vi "pco.camera_SaveImages_Example_IMAQ.vi"() -> ()   [LabVIEW 2020]
uses:
  <userlib>/PCO LabVIEW 5.0.0/pco.camera/Camera.lvclass
panel:
  out "rawImage":u16[][](array[numeric])
  out "Image":T1(plugin-control)
  in  "data_format":T2(ring)=enum."Mono16"
  in  "Image Index":u32 max=9
  in  "saveImages":bool
  in  "SavePath":path
  out "Recorded Images":u32
  in  "Quit":bool
  in  "roiY1":u64=2 min=2 max=2160 step=1
  in  "roiX1":u64=2 min=2 max=2560 step=1
  in  "roiY0":u64=1 min=1 max=2159 step=1
  in  "roiX0":u64=1 min=1 max=2559 step=1
  out "Image Height":u16
  out "Image Width":u16
  in  "dwImgCount":u32=10 caption="Required Number of Images" max=4023
  out "Error":errorcluster {"code" format="%x"}
  # "This example shows how to record an image sequence and save all images to files (and an .avi) afterwards.\nIt is a good starting point for writing own applications with file saving\nBut it will not be fail save, i.e. doesnt react on errors, just handles them forward to the end\n\nUsage:\nSelect your required image count you want to record before you start the program.\nOnce started, the camera class will be initialized and images will be recorded automatically.\nWhen acquisition has finished you can read the images by index, crop them using the ROI parameters and select a file path.\nBy clicking save, the images are saved with the selected file format using the current active roi setting.\nThis also finishes the program and will force an exit of the camera class"
  # "pco.labview"
  # "Camera Setup"
  # "Recording Control"
  # "Parameters for image readout"
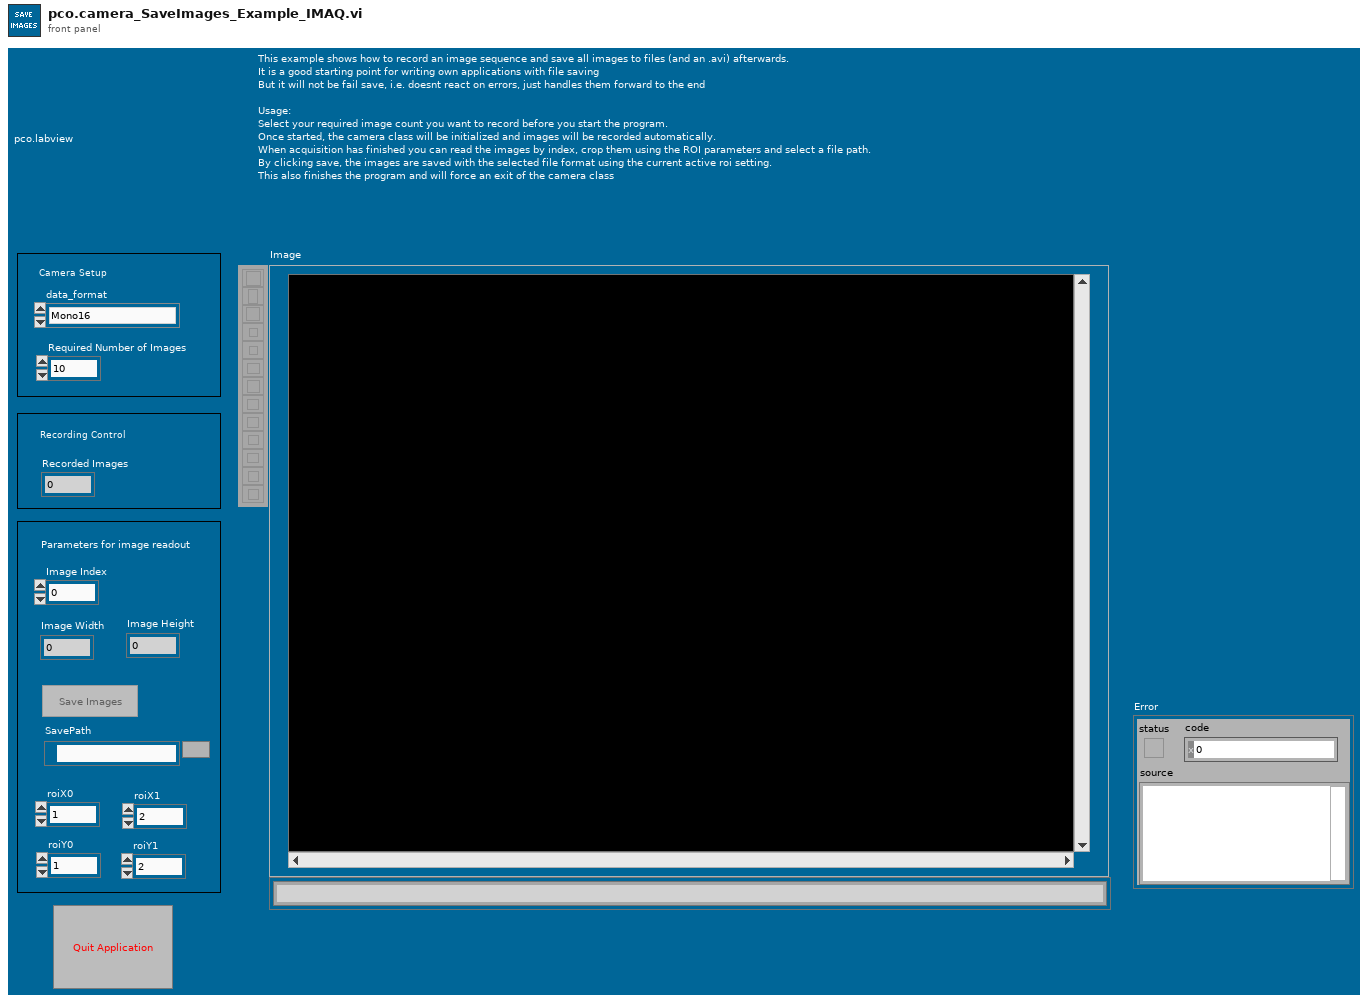
[diagram p1: front panel]
types:
  T1 = typedef "IMAQ Image.ctl" = refnum<image>
  T2 = enum16{"Undefined", "Mono8", "Mono16", "BGRA8", "RGBA8", "BGRA16", "RGBA16", "CompressedMono8"}
  T3 = enum8{"Enabled", "Disabled", "Disabled and Grayed Out"}
  T4 = enum16{"sequence", "sequence non blocking", "ring buffer", "fifo", "sequence_dpcore", "sequence_non_blocking_dpcore", "ring_buffer_dpcore", "fifo_dpcore", "tif", "multitif", "pcoraw", "b16", "dicom", "multidicom"}
  T5 = typedef "Image Type" = u32
  T6 = typedef "Camera.lvclass/binning.ctl" = cluster{"vert":u16, "horz":u16}
  T7 = cluster{"exposure_time_s":dbl, "delay_time_s":dbl, "roi":cluster{"x0":u64, "y0":u64, "x1":u64, "y1":u64}, "timestamp_mode":u16, "pixelrate":u32, "trigger_mode":u16, "acquire_mode":u16, "metadata_mode":u16, "noisefilter_mode":u16, "binning":T6}
  T8 = typedef "Color (U64)" = cluster{"Plane 3 (Blue)":u16, "Plane 2 (Green)":u16, "Plane 1 (Red)":u16, "Plane 4 (alpha)":u16}
  T9 = cluster{"dwImgCounter":u32, "lvTimestamp":timestamp, "dwMicroSeconds":u32}[]
  T10 = cluster{"dwImgCounter":u32, "lvTimestamp":timestamp, "dwMicroSeconds":u32}
  T11 = typedef "IMAQ AVI2 Refnum.ctl" = refnum<k20>
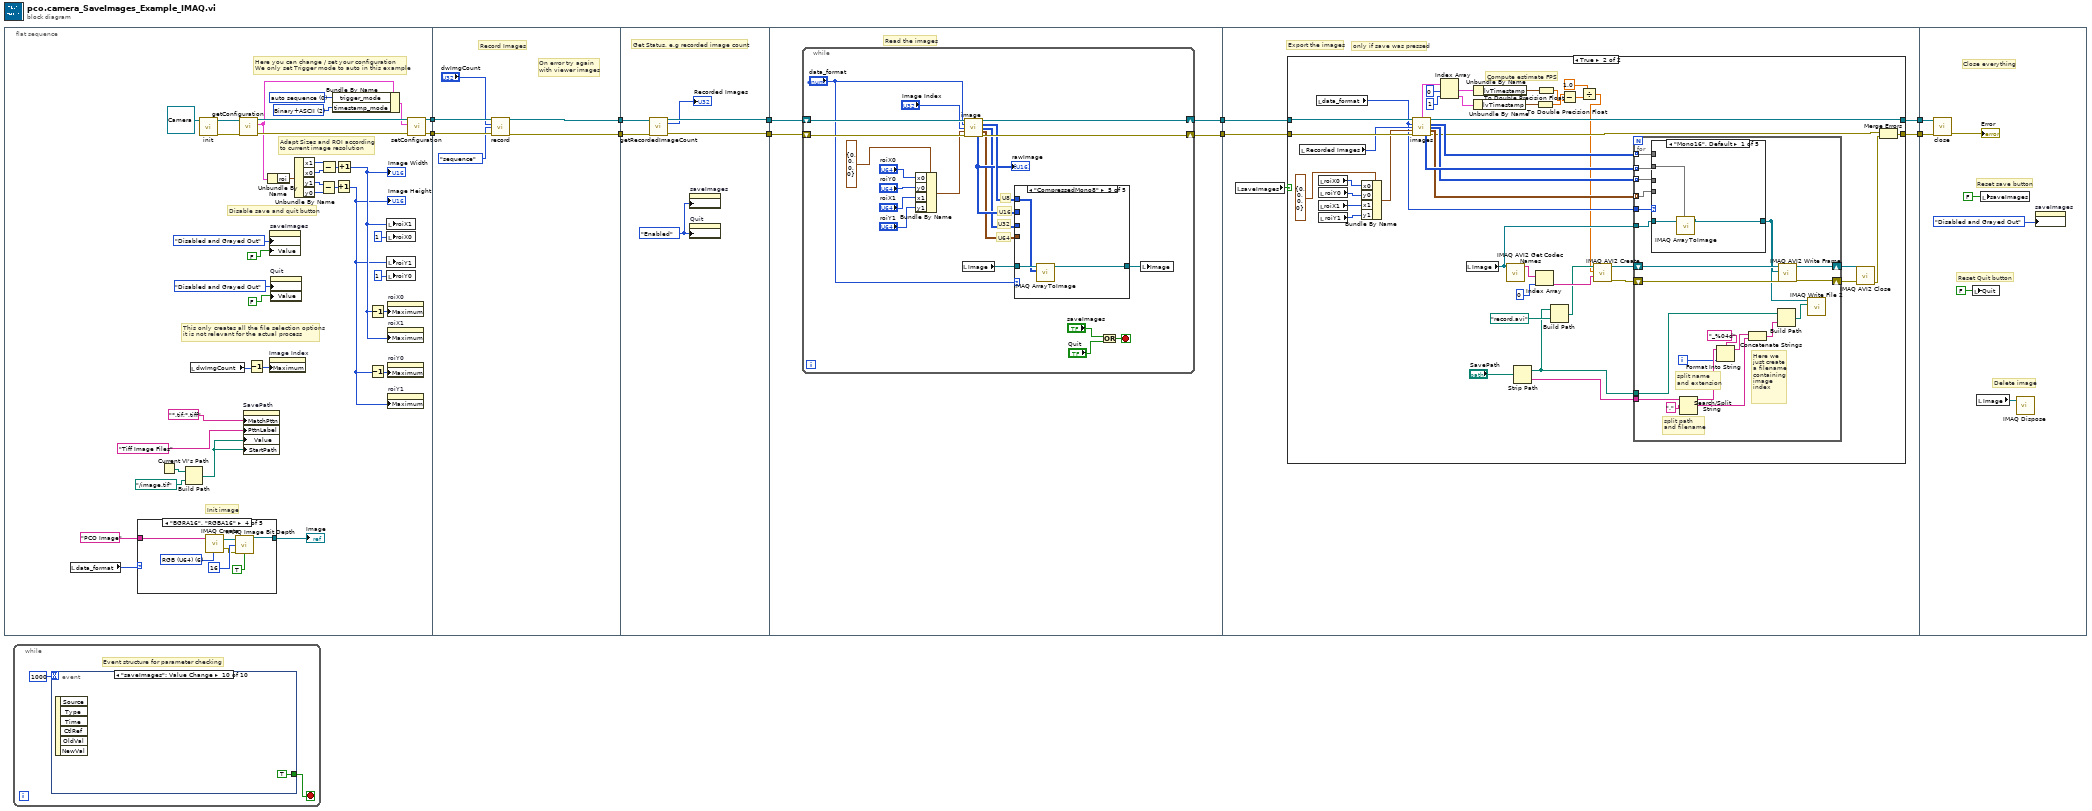
[diagram p0: block diagram]
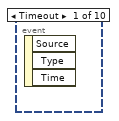
[diagram p2: hidden frame]
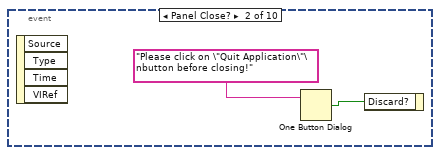
[diagram p3: hidden frame]
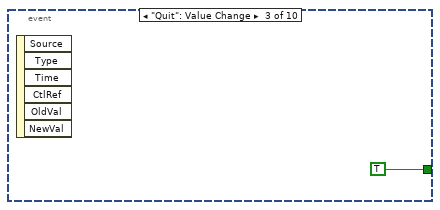
[diagram p4: hidden frame]
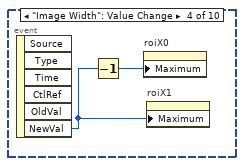
[diagram p5: hidden frame]
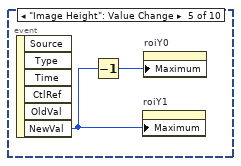
[diagram p6: hidden frame]
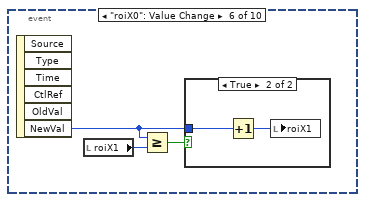
[diagram p7: hidden frame]
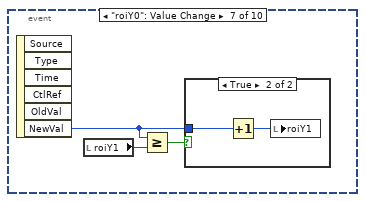
[diagram p9: hidden frame]
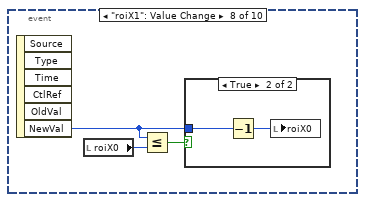
[diagram p11: hidden frame]
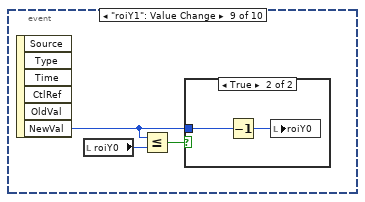
[diagram p13: hidden frame]
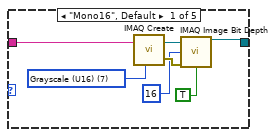
[diagram p15: hidden frame]
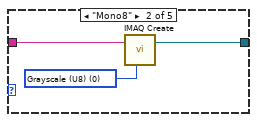
[diagram p16: hidden frame]
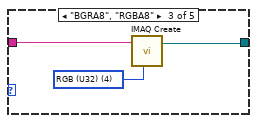
[diagram p17: hidden frame]
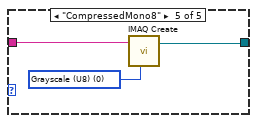
[diagram p18: hidden frame]
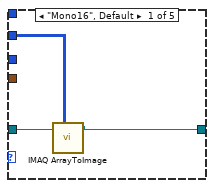
[diagram p19: hidden frame]
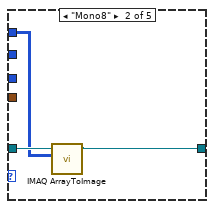
[diagram p20: hidden frame]
diagram:
  n1 = flat-sequence {
    tunnel: [w39] -> w10
    tunnel: [w38] -> w9
    tunnel: w10 -> [w77]
    tunnel: w9 -> [w76]
    tunnel: [w74] -> w8
    tunnel: [w73] -> w7
    tunnel: w8 -> [w83]
    tunnel: w7 -> [w82]
    tunnel: [w81] -> w6
    tunnel: [w80] -> w5
    tunnel: w6 -> [w86]
    tunnel: w5 -> [w87]
    tunnel: [w85] -> w4
    tunnel: [w84] -> w2
    tunnel: w4 -> [w127]
    tunnel: [w126] -> w3
    tunnel: w2 -> [w125]
    tunnel: [w124] -> w1
    tunnel: w3 -> [w216]
    tunnel: w1 -> [w215]
    frame #0 {
      w23 = u16 2 items=["OFF", "Binary", "Binary+ASCII", "ASCII"] ("TimestampMode")
      w45 = u16 0 items=["auto sequence"=0, "software trigger"=1, "external exposure start & software trigger"=2, "external exposure control"=3, "external synchronized"=4, "fast external exposure control"=5, "external CDS control"=6, "slow external exposure control"=7, "external synchronized HDSDI"=258] ("TriggerMode")
      # "Init image"
      # "This only creates all the file selection options\nit is not relevant for the actual process"
      # "Adapt Sizes and ROI according\nto current image resolution"
      # "Disable save and quit button"
      # "Here you can change / set your configuration\nWe only set Trigger mode to auto in this example"
      n2 = local read "data_format"() -> (w13:T2)
      n3 = case shown="\"BGRA16\", \"RGBA16\"" w13 {
        tunnel: "PCO Image" ("Image Name") -> [w54 w58 w60 w67 w70]
        tunnel: [w49 w56 w59 w64 w69] -> w12
        frame "Mono16", Default {
          w55 = T5 7 items=["Grayscale (U8)", "Grayscale (I16)", "Grayscale (SGL)", "Complex (CSG)", "RGB (U32)", "HSL (U32)", "RGB (U64)", "Grayscale (U16)"] ("Image Type")
          n4 = call "IMAQ Create"("Image Name"=w54, "Image Type"=w55) -> ("New Image"=w53:T1, "error out"=w52:errorcluster)  [unwired: 3 in]
          n5 = call "IMAQ Image Bit Depth"("Image"=w53, "Bit Depth (0)"=u32 16, "error in (no error)"=w52, "Get/Set Bit Depth? (Set)"=TRUE) -> ("Image Out"=w49:T1)  [unwired: 9 in, 2 out]
        }
        frame "Mono8" {
          w57 = T5 0 items=["Grayscale (U8)", "Grayscale (I16)", "Grayscale (SGL)", "Complex (CSG)", "RGB (U32)", "HSL (U32)", "RGB (U64)", "Grayscale (U16)"] ("Image Type")
          n6 = call "IMAQ Create"("Image Name"=w58, "Image Type"=w57) -> ("New Image"=w56:T1)  [unwired: 3 in, 1 out]
        }
        frame "BGRA8", "RGBA8" {
          w61 = T5 4 items=["Grayscale (U8)", "Grayscale (I16)", "Grayscale (SGL)", "Complex (CSG)", "RGB (U32)", "HSL (U32)", "RGB (U64)", "Grayscale (U16)"] ("Image Type")
          n7 = call "IMAQ Create"("Image Name"=w60, "Image Type"=w61) -> ("New Image"=w59:T1)  [unwired: 3 in, 1 out]
        }
        frame "BGRA16", "RGBA16" {
          w68 = T5 6 items=["Grayscale (U8)", "Grayscale (I16)", "Grayscale (SGL)", "Complex (CSG)", "RGB (U32)", "HSL (U32)", "RGB (U64)", "Grayscale (U16)"] ("Image Type")
          n8 = call "IMAQ Create"("Image Name"=w67, "Image Type"=w68) -> ("New Image"=w65:T1, "error out"=w62:errorcluster)  [unwired: 3 in]
          n9 = call "IMAQ Image Bit Depth"("Image"=w65, "Bit Depth (0)"=u32 16, "error in (no error)"=w62, "Get/Set Bit Depth? (Set)"=TRUE) -> ("Image Out"=w64:T1)  [unwired: 9 in, 2 out]
        }
        frame "CompressedMono8" {
          w71 = T5 0 items=["Grayscale (U8)", "Grayscale (I16)", "Grayscale (SGL)", "Complex (CSG)", "RGB (U32)", "HSL (U32)", "RGB (U64)", "Grayscale (U16)"] ("Image Type")
          n10 = call "IMAQ Create"("Image Name"=w70, "Image Type"=w71) -> ("New Image"=w69:T1)  [unwired: 3 in, 1 out]
        }
      }
      "Image" <- w12
      n11 = Current VI's Path() -> (path=w20:path)
      n12 = Build Path(base path=w20, name or relative path=path "../image.tif" ("SavePath")) -> (appended path=w17:path)
      n13 = local read "dwImgCount"() -> (w15:u32)
      n14 = call-dynamic "init.vi"("Camera in"=refnum<class "Camera.lvclass"> refnum ("PCOCamera in")) -> ("Camera out"=w47:refnum<class "Camera.lvclass">, "error out"=w46:errorcluster)  [unwired: 8 in]
      n15 = call-dynamic "getConfiguration.vi"("error in (no error)"=w46, "Camera in"=w47) -> ("error out"=w43:errorcluster, "configuration"=w33:T7, "Camera out"=w44:refnum<class "Camera.lvclass">)  [unwired: 7 in]
      n16 = property on="SavePath" class="Path"("MatchPttn"="*.tif;*.tiff" ("pattern (all files)"), "PttnLabel"="Tiff Image Files" ("pattern label"), "Value"=w17, "StartPath"=w17) -> ()  [unwired: 2 in, 2 out]
      n17 = Decrement(x=w15) -> (x-1=w16:u32)
      n18 = Unbundle By Name(w33) -> ("roi"=w32:cluster{"x0":u64, "y0":u64, "x1":u64, "y1":u64})
      n19 = property on="Image Index" class="DigNum (strict)"("Maximum"=w16) -> ()  [unwired: 2 in, 2 out]
      n20 = property on="saveImages" class="Bool (strict)"("DisabledEnum"=T3."Disabled and Grayed Out" ("Disabled"), "Value"=FALSE ("Stop")) -> ()  [unwired: 2 in, 2 out]
      n21 = property on="Quit" class="Bool (strict)"("DisabledEnum"=T3."Disabled and Grayed Out" ("Disabled"), "Value"=FALSE ("Stop")) -> ()  [unwired: 2 in, 2 out]
      n22 = Unbundle By Name(w32) -> ("x1"=w30:u64, "x0"=w31:u64, "y1"=w28:u64, "y0"=w29:u64)
      n23 = Subtract(x=w28, y=w29) -> (x-y=w26:u64)
      n24 = Subtract(x=w30, y=w31) -> (x-y=w27:u64)
      n25 = Bundle By Name(cluster=w33, "trigger_mode"=w45, "timestamp_mode"=w23) -> (w42:T7)
      n26 = Increment(x=w26) -> (x+1=w24:u64)
      "Image Height" <- w24
      n27 = Increment(x=w27) -> (x+1=w25:u64)
      "Image Width" <- w25
      n28 = Decrement(x=w25) -> (x-1=w35:u64)
      n29 = Decrement(x=w24) -> (x-1=w34:u64)
      n30 = local write "roiX1"(w25) -> ()
      n31 = local write "roiX0"(u16 1 ("roiY0")) -> ()
      n32 = local write "roiY1"(w24) -> ()
      n33 = local write "roiY0"(u16 1 ("roiY0")) -> ()
      n34 = property on="roiX0" class="DigNum (strict)"("Maximum"=w35) -> ()  [unwired: 2 in, 2 out]
      n35 = property on="roiX1" class="DigNum (strict)"("Maximum"=w25) -> ()  [unwired: 2 in, 2 out]
      n36 = property on="roiY0" class="DigNum (strict)"("Maximum"=w34) -> ()  [unwired: 2 in, 2 out]
      n37 = property on="roiY1" class="DigNum (strict)"("Maximum"=w24) -> ()  [unwired: 2 in, 2 out]
      n38 = call-dynamic "setConfiguration.vi"("error in (no error)"=w43, "configuration"=w42, "Camera in"=w44) -> ("error out"=w38:errorcluster, "Camera out"=w39:refnum<class "Camera.lvclass">)  [unwired: 7 in]
    }
    frame #1 {
      # "On error try again \nwith viewer images"
      # "Record Images"
      n39 = call-dynamic "record.vi"("Camera in"=w77, "num_images"="dwImgCount", "record_mode"=T4."sequence", "error in (no error)"=w76) -> ("Camera out"=w74:refnum<class "Camera.lvclass">, "error out"=w73:errorcluster)  [unwired: 10 in]
    }
    frame #2 {
      w78 = T3."Enabled" ("Disabled")
      # "Get Status, e.g recorded image count"
      n40 = call-dynamic "getRecordedImageCount.vi"("Camera in"=w83, "error in (no error)"=w82) -> ("Camera out"=w81:refnum<class "Camera.lvclass">, "recorded_image_count"=→"Recorded Images":u32, "error out"=w80:errorcluster)  [unwired: 11 in]
      n41 = property on="saveImages" class="Bool (strict)"("DisabledEnum"=w78) -> ()  [unwired: 2 in, 2 out]
      n42 = property on="Quit" class="Bool (strict)"("DisabledEnum"=w78) -> ()  [unwired: 2 in, 2 out]
    }
    frame #3 {
      # "Read the images"
      n43 = while {
        shift-right: [w106] -> w85
        shift-left: w86 -> [w108]
        shift-right: [w101] -> w84
        shift-left: w87 -> [w107]
        stop <- w99 stop-if-true
        # "U64"
        # "U32"
        # "U16"
        # "U8"
        n44 = Bundle By Name(cluster=cluster{"x0":u64, "y0":u64, "x1":u64, "y1":u64} {"x0"=0, "y0"=0, "x1"=0, "y1"=0} ("roi"), "x0"="roiX0", "y0"="roiY0", "x1"="roiX1", "y1"="roiY1") -> (w97:cluster{"x0":u64, "y0":u64, "x1":u64, "y1":u64})
        n45 = local read "Image"() -> (w90:T1)
        n46 = call-dynamic "image.vi"("Camera in"=w108, "data_format"="data_format", "image_index"="Image Index", "roi"=w97, "error in (no error)"=w107) -> ("Camera out"=w106:refnum<class "Camera.lvclass">, "image (U8)"=w94:u8[][], "image (U32)"=w92:u32[][], "image (U64)"=w91:T8[][], "raw_image (U16)"=w93:u16[][], "error out"=w101:errorcluster)  [unwired: 3 in, 2 out]
        "rawImage" <- w93
        n47 = case shown="\"CompressedMono8\"" "data_format" {
          tunnel: w90 -> [w111 w114 w117 w120 w123]
          tunnel: [w109 w112 w116 w118 w122] -> w89
          tunnel: w91 -> [_ _ _ w119 _]
          tunnel: w92 -> [_ _ w115 _ _]
          tunnel: w94 -> [_ w113 _ _ w121]
          tunnel: w93 -> [w110 _ _ _ _]
          frame "Mono16", Default {
            n48 = call "IMAQ ArrayToImage"("Image Pixels (U16)"=w110, "Image"=w111) -> ("Image Out"=w109:T1)  [unwired: 8 in, 1 out]
          }
          frame "Mono8" {
            n49 = call "IMAQ ArrayToImage"("Image Pixels (U8)"=w113, "Image"=w114) -> ("Image Out"=w112:T1)  [unwired: 8 in, 1 out]
          }
          frame "BGRA8", "RGBA8" {
            n50 = call "IMAQ ArrayToColorImage"("Image Pixels (U32)"=w115, "Image"=w117) -> ("Image Out"=w116:T1)  [unwired: 3 in, 1 out]
          }
          frame "BGRA16", "RGBA16" {
            n51 = call "IMAQ ArrayToColorImage"("Image"=w120, "Image Pixels (U64)"=w119) -> ("Image Out"=w118:T1)  [unwired: 3 in, 1 out]
          }
          frame "CompressedMono8" {
            n52 = call "IMAQ ArrayToImage"("Image Pixels (U8)"=w121, "Image"=w123) -> ("Image Out"=w122:T1)  [unwired: 8 in, 1 out]
          }
        }
        n53 = Or(x="saveImages", y="Quit") -> (x .or. y?=w99:bool)
        n54 = local write "Image"(w89) -> ()
      }
    }
    frame #4 {
      # "only if save was pressed"
      # "Export the images"
      n55 = local read "saveImages"() -> (w128:bool)
      n56 = case shown="True" w128 {
        tunnel: w127 -> [w130 w172]
        tunnel: [w130 w157] -> w126
        tunnel: w125 -> [w129 w173]
        tunnel: [w129 w150] -> w124
        frame False {
        }
        frame True {
          # "Compute estimate FPS"
          n57 = local read "Recorded Images"() -> (w165:u32)
          n58 = local read "data_format"() -> (w148:T2)
          n59 = local read "roiX0"() -> (w170:u64)
          n60 = local read "roiX1"() -> (w168:u64)
          n61 = local read "roiY0"() -> (w169:u64)
          n62 = local read "roiY1"() -> (w167:u64)
          n63 = Bundle By Name(cluster=cluster{"x0":u64, "y0":u64, "x1":u64, "y1":u64} {"x0"=0, "y0"=0, "x1"=0, "y1"=0} ("roi"), "x0"=w170, "y0"=w169, "x1"=w168, "y1"=w167) -> (w166:cluster{"x0":u64, "y0":u64, "x1":u64, "y1":u64})
          n64 = call-dynamic "images.vi"("Camera in"=w172, "data_format"=w148, "image_count"=w165, "roi"=w166, "error in (no error)"=w173) -> ("timestamp_list"=w142:T9, "Camera out"=w157:refnum<class "Camera.lvclass">, "image_list (U8)"=w161:u8[][][], "image_list (U32)"=w159:u32[][][], "image_list (U64)"=w158:T8[][][], "raw_image_list (U16)"=w160:u16[][][], "error out"=w152:errorcluster)  [unwired: 3 in, 1 out]
          n65 = Index Array(array=w142, index #1=0 ("index"), index #2=1 ("index")) -> (element #1=w139:T10, element #2=w138:T10)
          n66 = local read "Image"() -> (w149:T1)
          n67 = Unbundle By Name(w138) -> ("lvTimestamp"=w136:timestamp)
          n68 = Unbundle By Name(w139) -> ("lvTimestamp"=w137:timestamp)
          n69 = call "IMAQ AVI2 Get Codec Names"("Image"=w149) -> ("Codec Names"=w164:string[])  [unwired: 9 in, 1 out]
          n70 = Strip Path(path="SavePath") -> (stripped path=w143:path, name=w146:string)
          n71 = Index Array(array=w164, index=0) -> (element=w162:string)
          n72 = To Double Precision Float(number=w136) -> (double precision float=w135:dbl)
          n73 = To Double Precision Float(number=w137) -> (double precision float=w134:dbl)
          n74 = Build Path(base path=w143, name or relative path=path "record.avi") -> (appended path=w144:path)
          n75 = Subtract(x=w135, y=w134) -> (x-y=w133:dbl)
          n76 = Divide(x=1.0, y=w133) -> (x/y=w131:dbl)
          n77 = call "IMAQ AVI2 Create"("Codec"=w162, "Frames Per Second"=w131, "AVI Path"=w144) -> ("error out"=w156:errorcluster, "AVI Refnum"=w155:T11)  [unwired: 7 in]
          n78 = for {
            tunnel: w161 -> [w194] mode=indexing
            tunnel: w160 -> [w193] mode=indexing
            tunnel: w159 -> [w192] mode=indexing
            tunnel: w158 -> [w191] mode=indexing
            shift-right: [w187] -> w153
            shift-left: w155 -> [w190]
            shift-right: [w188] -> w154
            shift-left: w156 -> [w189]
            tunnel: w149 -> [w177]
            tunnel: w148 -> [w176]
            tunnel: w146 -> [w175]
            tunnel: w143 -> [w174]
            i -> [w179]
            # "Here we \njust create\na filename\ncontaining\nimage \nindex"
            # "split path \nand filename"
            # "split name \nand extension"
            n79 = case shown="\"Mono16\", Default" w176 {
              tunnel: w177 -> [w197 w200 w203 w206 w209]
              tunnel: [w195 w198 w202 w204 w208] -> w186
              tunnel: w191 -> [_ _ _ w205 _]
              tunnel: w192 -> [_ _ w201 _ _]
              tunnel: w194 -> [_ w199 _ _ w207]
              tunnel: w193 -> [w196 _ _ _ _]
              frame "Mono16", Default {
                n80 = call "IMAQ ArrayToImage"("Image Pixels (U16)"=w196, "Image"=w197) -> ("Image Out"=w195:T1)  [unwired: 8 in, 1 out]
              }
              frame "Mono8" {
                n81 = call "IMAQ ArrayToImage"("Image Pixels (U8)"=w199, "Image"=w200) -> ("Image Out"=w198:T1)  [unwired: 8 in, 1 out]
              }
              frame "BGRA8", "RGBA8" {
                n82 = call "IMAQ ArrayToColorImage"("Image Pixels (U32)"=w201, "Image"=w203) -> ("Image Out"=w202:T1)  [unwired: 3 in, 1 out]
              }
              frame "BGRA16", "RGBA16" {
                n83 = call "IMAQ ArrayToColorImage"("Image"=w206, "Image Pixels (U64)"=w205) -> ("Image Out"=w204:T1)  [unwired: 3 in, 1 out]
              }
              frame "CompressedMono8" {
                n84 = call "IMAQ ArrayToImage"("Image Pixels (U8)"=w207, "Image"=w209) -> ("Image Out"=w208:T1)  [unwired: 8 in, 1 out]
              }
            }
            n85 = Search/Split String(string=w175, search string/char (-)=".") -> (substring before match=w183:string, match + rest of string=w184:string)  [unwired: 1 in, 1 out]
            n86 = Format Into String(format string="_%04d", initial string=w183, w179) -> (resulting string=w185:string)  [unwired: 1 in, 1 out]
            n87 = Concatenate Strings(w185, w184) -> (w180:string)
            n88 = Build Path(base path=w174, name or relative path=w180) -> (appended path=w178:path)
            n89 = call "IMAQ AVI2 Write Frame"("error in (no error)"=w189, "Image"=w186, "AVI Refnum"=w190) -> ("error out"=w188:errorcluster, "AVI Refnum (duplicate)"=w187:T11)  [unwired: 6 in, 1 out]
            n90 = call-poly "IMAQ Write File 2"("File Path"=w178, "Image"=w186) -> ()  [unwired: 8 in, 2 out]
          }
          n91 = call "IMAQ AVI2 Close"("error in (no error)"=w154, "AVI Refnum"=w153) -> ("error out"=w151:errorcluster)  [unwired: 9 in]
          n92 = Merge Errors(w152, w151) -> (w150:errorcluster)
        }
      }
    }
    frame #5 {
      # "Delete image"
      # "Reset Quit button"
      # "Close everything"
      # "Reset save button"
      n93 = call-dynamic "close.vi"("error in (no error)"=w215, "Camera in"=w216) -> ("error out"=→"Error":errorcluster)  [unwired: 9 in]
      n94 = local write "Quit"(FALSE ("Stop")) -> ()
      n95 = local read "Image"() -> (w210:T1)
      n96 = local write "saveImages"(FALSE ("Stop")) -> ()
      n97 = call "IMAQ Dispose"("Image"=w210) -> ()  [unwired: 5 in, 1 out]
      n98 = property on="saveImages" class="Bool (strict)"("DisabledEnum"=T3."Disabled and Grayed Out" ("Disabled")) -> ()  [unwired: 2 in, 2 out]
    }
  }
  n99 = while {
    stop <- w217 stop-if-true
    # "Event structure for parameter checking"
    n100 = event shown="[9] \"saveImages\": Value Change" {
      selector: _ -> [_ _ _ _ _ _ _ _ _ _]
      dyn-events: _ -> [_ _ _ _ _ _ _ _ _ _]
      timeout: 1000 -> [_ _ _ _ _ _ _ _ _ _]
      tunnel: [_ _ TRUE _ _ _ _ _ _ TRUE] -> w217
      event Timeout {
        n101 = event-data() -> ()  [unwired: 1 in, 3 out]
      }
      event Panel Close? {
        n102 = event-data() -> ()  [unwired: 1 in, 4 out]
        n103 = One Button Dialog(message="Please click on \"Quit Application\"\nbutton before closing!") -> (true=w219:bool)  [unwired: 1 in]
        n104 = event-data("Discard?"=w219) -> ()  [unwired: 1 in, 1 out]
      }
      event "Quit": Value Change {
        n105 = event-data() -> ()  [unwired: 1 in, 6 out]
      }
      event "Image Width": Value Change {
        n106 = event-data() -> ("NewVal"=w222:u16)  [unwired: 1 in, 5 out]
        n107 = Decrement(x=w222) -> (x-1=w223:u16)
        n108 = property on="roiX0" class="DigNum (strict)"("Maximum"=w223) -> ()  [unwired: 2 in, 2 out]
        n109 = property on="roiX1" class="DigNum (strict)"("Maximum"=w222) -> ()  [unwired: 2 in, 2 out]
      }
      event "Image Height": Value Change {
        n110 = event-data() -> ("NewVal"=w224:u16)  [unwired: 1 in, 5 out]
        n111 = Decrement(x=w224) -> (x-1=w225:u16)
        n112 = property on="roiY1" class="DigNum (strict)"("Maximum"=w224) -> ()  [unwired: 2 in, 2 out]
        n113 = property on="roiY0" class="DigNum (strict)"("Maximum"=w225) -> ()  [unwired: 2 in, 2 out]
      }
      event "roiX0": Value Change {
        n114 = event-data() -> ("NewVal"=w226:u64)  [unwired: 1 in, 5 out]
        n115 = local read "roiX1"() -> (w228:u64)
        n116 = Greater Or Equal?(x=w226, y=w228) -> (x >= y?=w227:bool)
        n117 = case shown="True" w227 {
          tunnel: w226 -> [_ w230]
          frame False {
          }
          frame True {
            n118 = Increment(x=w230) -> (x+1=w229:u64)
            n119 = local write "roiX1"(w229) -> ()
          }
        }
      }
      event "roiY0": Value Change {
        n120 = event-data() -> ("NewVal"=w231:u64)  [unwired: 1 in, 5 out]
        n121 = local read "roiY1"() -> (w233:u64)
        n122 = Greater Or Equal?(x=w231, y=w233) -> (x >= y?=w232:bool)
        n123 = case shown="True" w232 {
          tunnel: w231 -> [_ w235]
          frame False {
          }
          frame True {
            n124 = Increment(x=w235) -> (x+1=w234:u64)
            n125 = local write "roiY1"(w234) -> ()
          }
        }
      }
      event "roiX1": Value Change {
        n126 = event-data() -> ("NewVal"=w236:u64)  [unwired: 1 in, 5 out]
        n127 = local read "roiX0"() -> (w238:u64)
        n128 = Less Or Equal?(x=w236, y=w238) -> (x <= y?=w237:bool)
        n129 = case shown="True" w237 {
          tunnel: w236 -> [_ w240]
          frame False {
          }
          frame True {
            n130 = Decrement(x=w240) -> (x-1=w239:u64)
            n131 = local write "roiX0"(w239) -> ()
          }
        }
      }
      event "roiY1": Value Change {
        n132 = event-data() -> ("NewVal"=w241:u64)  [unwired: 1 in, 5 out]
        n133 = local read "roiY0"() -> (w243:u64)
        n134 = Less Or Equal?(x=w241, y=w243) -> (x <= y?=w242:bool)
        n135 = case shown="True" w242 {
          tunnel: w241 -> [_ w245]
          frame False {
          }
          frame True {
            n136 = Decrement(x=w245) -> (x-1=w244:u64)
            n137 = local write "roiY0"(w244) -> ()
          }
        }
      }
      event "saveImages": Value Change {
        n138 = event-data() -> ()  [unwired: 1 in, 6 out]
      }
    }
  }
